vi "Downhill simplex formula string.vi"(5 "X":string[](array[string]), 7 "f(X)":string, 8 "error in (no error)":errorcluster, 9 "stopping criteria":T1={"function tolerance"=1e-06, "parameter tolerance"=1e-06, "max iterations"=100, "max function calls"=1000, "gradient tolerance"=1e-06, "max time (sec)"=-1.0}, 11 "start":dbl[](array[numeric])) -> (0 "error out":errorcluster, 1 "number of function evaluations":i32, 2 "f(minimum)":dbl, 3 "minimum":dbl[](array[numeric]))   [LabVIEW 2020, in "NI_Gmath.lvlib"]
doc: "Solves the unconstrained minimization problem for an arbitrary nonlinear function. You must manually select the polymorphic instance to use."
uses:
  <vilib>/gmath/NI_Gmath.lvlib
  <vilib>/gmath/NumericalOptimization/stopping criteria.ctl
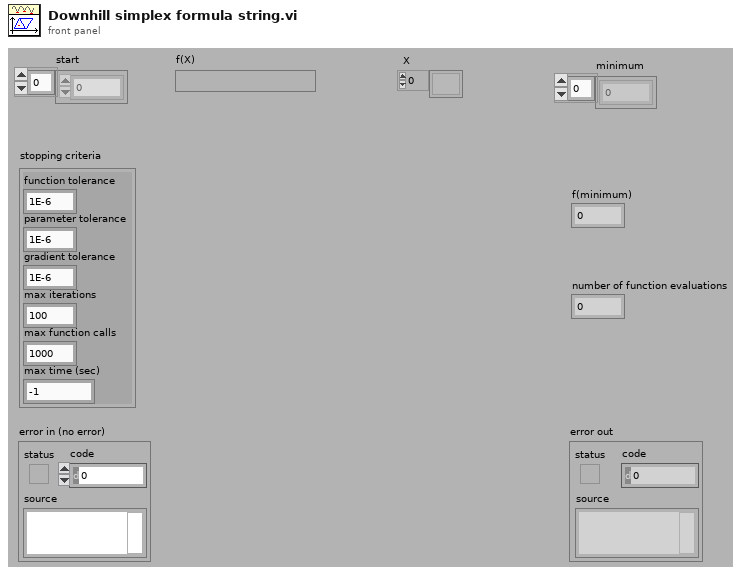
[diagram p1: front panel]
types:
  T1 = typedef "NI_Gmath.lvlib/stopping criteria.ctl" = cluster{"function tolerance":dbl, "parameter tolerance":dbl, "max iterations":i32, "max function calls":i32, "gradient tolerance":dbl, "max time (sec)":dbl}
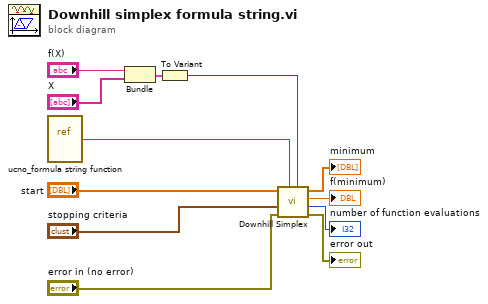
[diagram p0: block diagram]
diagram:
  n1 = vi-ref <vilib>:"ucno_formula string function.vi"() -> ("vi reference"=w3:refnum<vi>)
  n2 = Bundle("f(X)"="f(X)", "X"="X") -> (w5:cluster{"f(X)":string, "X":string[]})  [unwired: 1 in]
  n3 = To Variant(anything=w5) -> (Variant=w2:variant)
  n4 = call <vilib>:"Downhill Simplex.vi"("function data"=w2, "objective function"=w3, "error in (no error)"="error in (no error)", "stopping criteria"="stopping criteria", "start"="start") -> ("error out"=→"error out":errorcluster, "number of function evaluations"=→"number of function evaluations":i32, "f(minimum)"=→"f(minimum)":dbl, "minimum"=→"minimum":dbl[])  [unwired: 3 in]
